vi "Fit Transform.vi"(7 "Type X":T2(ring), 8 "error in (no error)":errorcluster caption="entrée d'erreur (pas d'erreur)", 9 "y":string[][](array[string]), 10 "X":string[][](array[string]), 11 "Nystroem.lvclass":refnum<class "Nystroem.lvclass">) -> (0 "error out":errorcluster caption="sortie d'erreur", 2 "Data":T1, 3 "Nystroem.lvclass":refnum<class "Nystroem.lvclass">)   [LabVIEW 2020, in "Nystroem.lvclass"]
doc: "Fit to data, then transform it.\n\nFits transformer to X and y with optional parameters fit_params and returns a transformed version of X.\n\nReturns : \n\n- X_new : ndarray array of shape (n_samples, n_features_new)\nTransformed array."
uses:
  Nystroem.lvclass
  Nystroem.lvclass/Nystroem.ctl
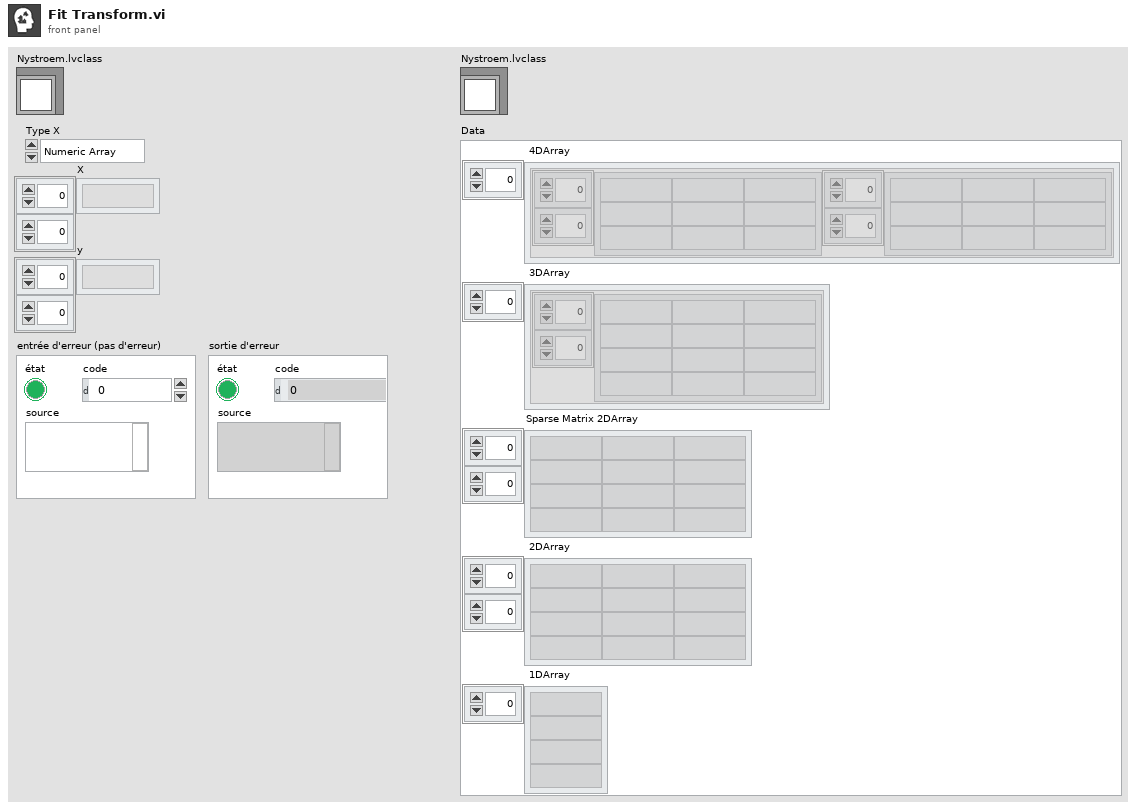
[diagram p1: front panel]
types:
  T1 = cluster{" 4DArray":cluster{"1":string[][], "2":string[][]}[], " 3DArray":cluster{"Tableau":string[][]}[], "Sparse Matrix 2DArray":string[][], " 2DArray":string[][], " 1DArray":string[]}
  T2 = enum16{"Numeric Array", "String Array", "Sparse"}
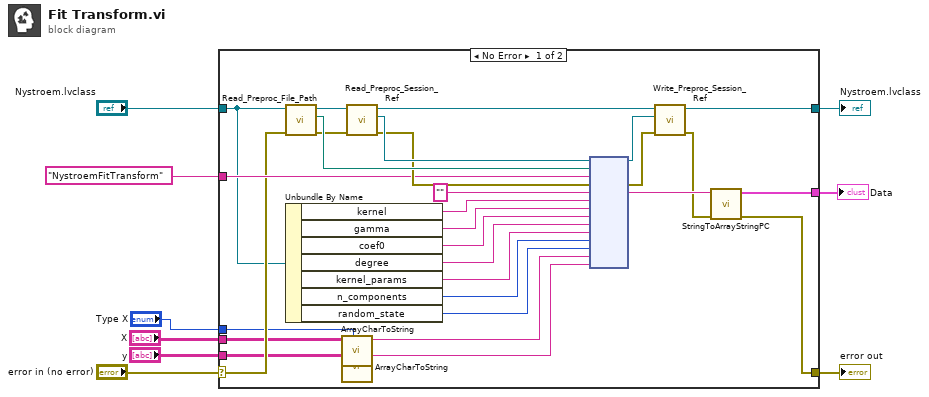
[diagram p0: block diagram]
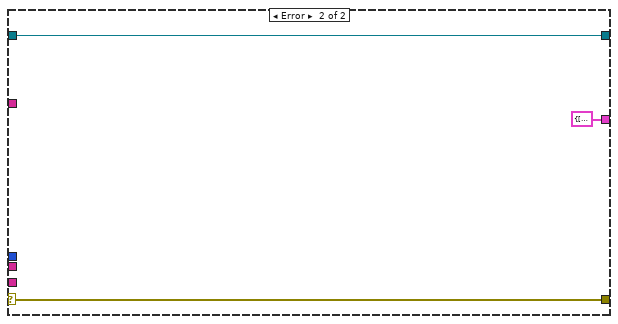
[diagram p2: hidden frame]
diagram:
  n1 = case shown="No Error" "error in (no error)" {
    selector: "error in (no error)" -> [w26 w41]
    tunnel: [w11 w41] -> w8
    tunnel: [w14 w40] -> w6
    tunnel: "Nystroem.lvclass" -> [w25 w40]
    tunnel: "NystroemFitTransform" ("Fonction") -> [w27 _]
    tunnel: "X" -> [w19 _]
    tunnel: "y" -> [w16 _]
    tunnel: "Type X" -> [w17 _]
    tunnel: [w10 T1 {" 4DArray"=[], " 3DArray"=[], "Sparse Matrix 2DArray"=[], " 2DArray"=[], " 1DArray"=[]} ("Data")] -> w1
    frame No Error {
      n2 = call-dynamic "Read_Preproc_File_Path.vi"("error in (no error)"=w26, "Python in"=w25) -> ("error out"=w33:errorcluster, "File_Path"=w36:path, "Python out"=w38:refnum<class "Nystroem.lvclass">)  [unwired: 7 in]
      n3 = Unbundle By Name(w25) -> ("kernel"=w29:string, "gamma"=w28:string, "coef0"=w24:string, "degree"=w23:string, "kernel_params"=w22:string, "n_components"=w21:i32, "random_state"=w20:i32)
      n4 = call "ArrayCharToString.vi"("Type"=w17, "TAB"=w19) -> ("Instruction"=w18:string)  [unwired: 9 in]
      n5 = call "ArrayCharToString.vi"("TAB"=w16) -> ("Instruction"=w15:string)  [unwired: 10 in]
      n6 = call-dynamic "Read_Preproc_Session_Ref.vi"("error in (no error)"=w33, "Python in"=w38) -> ("error out"=w34:errorcluster, "Session_ref"=w35:refnum<k35>, "Python out"=w37:refnum<class "Nystroem.lvclass">)  [unwired: 7 in]
      n7 = node(w35, w36, w27, w34, "", w29, w28, w24, w23, w22, w21, w20, w18, w15) -> (w30:refnum<k35>, w32:errorcluster, w13:string)  [unwired: 9 in, 2 out]
      n8 = call-dynamic "Write_Preproc_Session_Ref.vi"("error in (no error)"=w32, "Session_ref"=w30, "Python in"=w37) -> ("error out"=w12:errorcluster, "Python out"=w14:refnum<class "Nystroem.lvclass">)  [unwired: 7 in]
      n9 = call "StringToArrayStringPC.vi"("sortie d'erreur"=w12, "Return value"=w13) -> ("sortie d'erreur"=w11:errorcluster, "Data"=w10:T1)  [unwired: 8 in]
    }
    frame Error {
    }
  }
  "error out" <- w8
  "Nystroem.lvclass" <- w6
  "Data" <- w1
